vi "Calculate_Motor_Value.vi"(1 "Arm Direction":i16) -> (0 "Final Speed":dbl)   [LabVIEW 2012]
panel:
  in  "Motor Speed":dbl
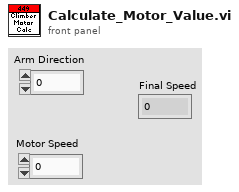
[diagram p1: front panel]
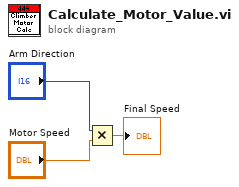
[diagram p0: block diagram]
diagram:
  n1 = Multiply(x="Arm Direction", y="Motor Speed") -> (x*y=→"Final Speed":dbl)
